vi "Actor Core.vi"(8 "error in":errorcluster, 11 "CrossPoint in":refnum<class "CrossPoint.lvclass">) -> (0 "error out":errorcluster, 3 "Actor out":refnum<class "Actor.lvclass">)   [LabVIEW 2019, in "CrossPoint.lvlib" / "CrossPoint.lvclass"]
doc: "The instrument actor core is only here to distribute panel resolution settings to children classes."
uses:
  Library/CrossPoint.lvclass
  builds/Engine/Actor Framework.lvlibp/1abvi3w/vi.lib/ActorFramework/Actor/Actor.lvclass
  builds/Instruments/Instruments.lvlibp/Library/Instruments.lvclass
  C:/Users/Public/Documents/Development/builds/Instruments/Instruments.lvlibp/Library/Instruments.lvclass
panel:
  in  "Clear All Routes":bool
  in  "Active Device":u16(ring)
  in  "Clear Selected Route":bool
  in  "Route Low Side":bool
  in  "Route High Side":bool
  in  "Measurement_Points":i32(listbox)
  in  "Instrument Low Side":i32(listbox)
  in  "Instrument High Side":i32(listbox)
  in  "Active Routes":i32(listbox)
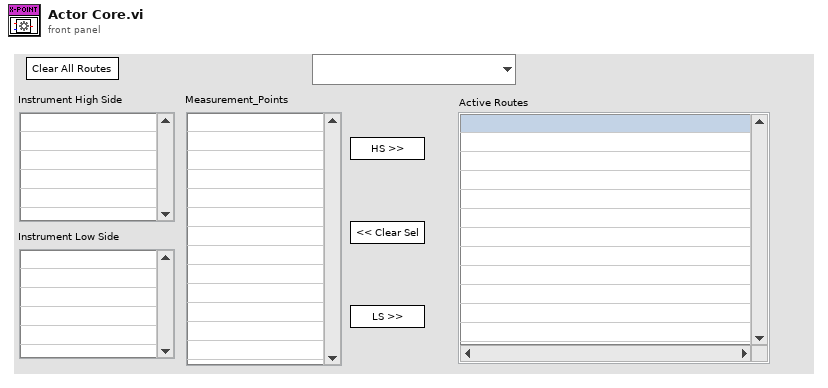
[diagram p1: front panel]
types:
  T1 = cluster{"Pnl Actor":refnum<event-registration>, "Event Registration Refnum":refnum<event-registration>}
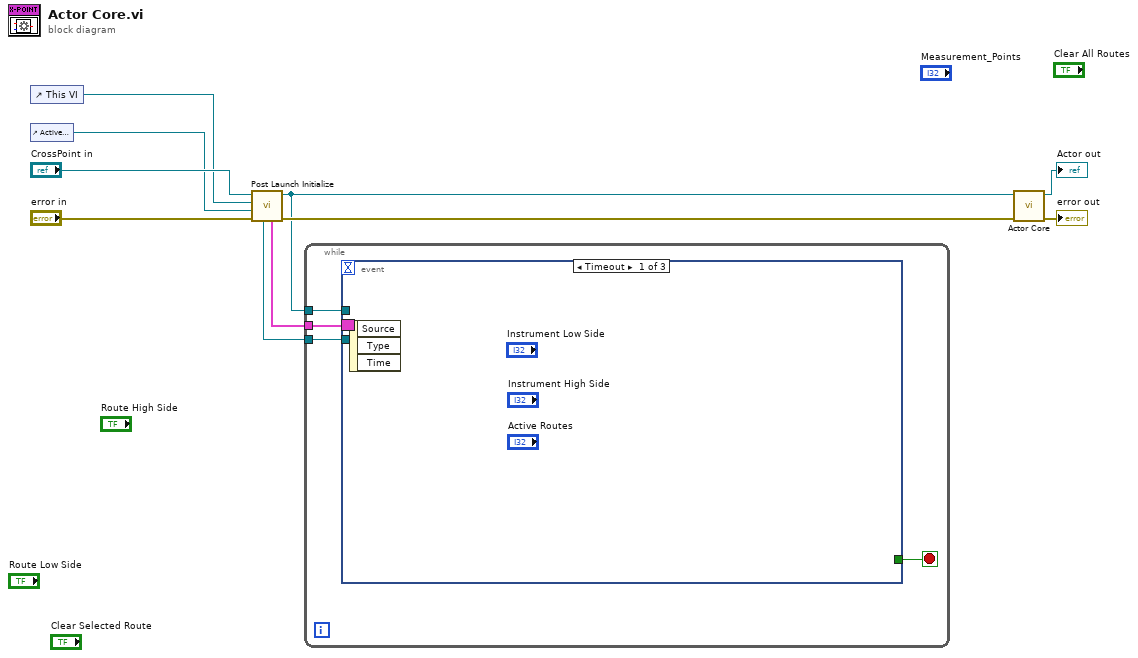
[diagram p0: block diagram]
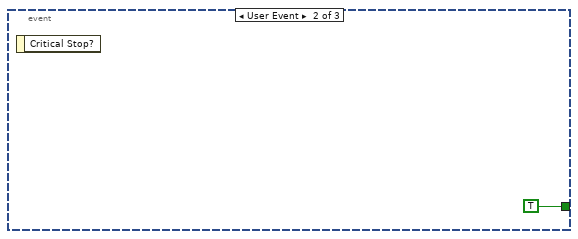
[diagram p2: hidden frame]
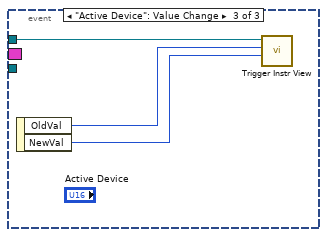
[diagram p3: hidden frame]
diagram:
  n1 = control-ref of="This VI"() -> (w5:refnum<vi>)
  n2 = control-ref of="Active Device"() -> (w4:refnum<vi>)
  n3 = call "Post Launch Initialize.vi"("error in"="error in", "Active Device"=w4, "GUI Reference"=w5, "Instruments in"="CrossPoint in") -> ("error out"=w7:errorcluster, "Instruments out"=w2:refnum<class "CrossPoint.lvclass">, "Registered Events"=w3:T1, "Self Enqueuer"=w1:refnum<class "Message Enqueuer.lvclass">)  [unwired: 4 in]
  n4 = while {
    tunnel: w3 -> [w14]
    tunnel: w2 -> [w13]
    tunnel: w1 -> [w12]
    stop <- w11 stop-if-true
    n5 = event shown="[0] Timeout" {
      selector: w14 -> [_ _ _]
      dyn-events: _ -> [_ _ _]
      timeout: _ -> [_ _ _]
      tunnel: w13 -> [_ _ w18]
      tunnel: w12 -> [_ _ _]
      tunnel: [_ TRUE _] -> w11
      event Timeout {
        n6 = event-data() -> ()  [unwired: 1 in, 3 out]
      }
      event User Event {
        n7 = event-data() -> ()  [unwired: 1 in, 1 out]
      }
      event "Active Device": Value Change {
        n8 = event-data() -> ("OldVal"=w17:u16, "NewVal"=w16:u16)  [unwired: 1 in]
        n9 = call "Trigger Instr View.vi"("New Value"=w16, "Old Value"=w17, "Instruments in"=w18) -> ()  [unwired: 7 in, 2 out]
      }
    }
  }
  n10 = call-parent "Actor Core.vi"("error in"=w7, "Instruments in"=w2) -> ("error out"=→"error out":errorcluster, "Actor out"=→"Actor out":refnum<class "Actor.lvclass">)  [unwired: 8 in]
